vi "Pre-Build Action.vi"(6 "Top Level/Always Included VIs":path[](array[path]), 7 "Main Destination Path":path, 9 "Target Name":string, 10 "Build Specification Name":string, 11 "Project Path":path) -> (0 "error out":errorcluster)   [LabVIEW 2020]
doc: "Get all of the VIPM packages installed in the machine and modify the constant array value to list all installed VIPM packages."
uses:
  <vilib>/JKI/VIPM API/VIPM API_vipm_api.lvlib
panel:
  # "Overview: Get all of the VIPM packages installed in the machine and modify the constant array value to list all installed VIPM packages.\nRequirements: Target VI\nInstructions:\n1. (#TODO1) In the block diagram, specify the target VI reference\n2. (#TODO2) Specify the label name like this in the target VI\nor change the string constant in the block diagram to make it the same as the constant label in the target VI\n(Note: the constant must be 1D String Array)\n3. (#TODO3) Replace the included control/indicator with your orginal control/indicator if you're using the pre-built VI template \n3. Set this VI as Pre Build in the project Build Specifications Properties (Pre/Post Build Actions -> Execute VI before build)"
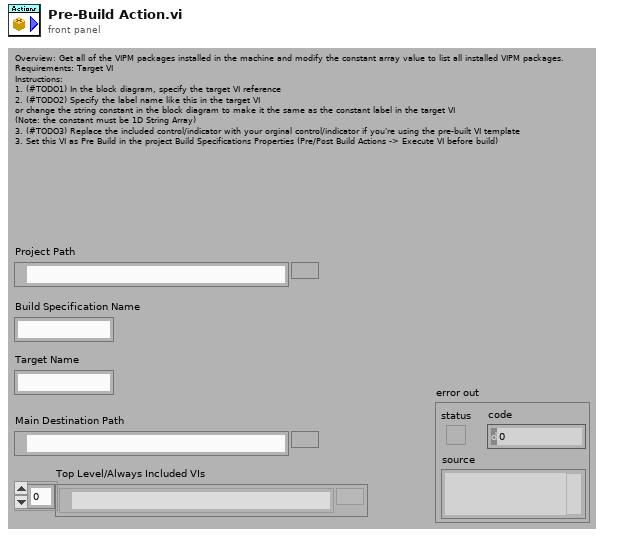
[diagram p1: front panel]
types:
  T1 = typedef "VIPM API_vipm_api.lvlib/LabVIEW Target Info Cluster_vipm_api.ctl" = cluster{"Version":string, "Connection Tested":bool, "Disabled":bool}
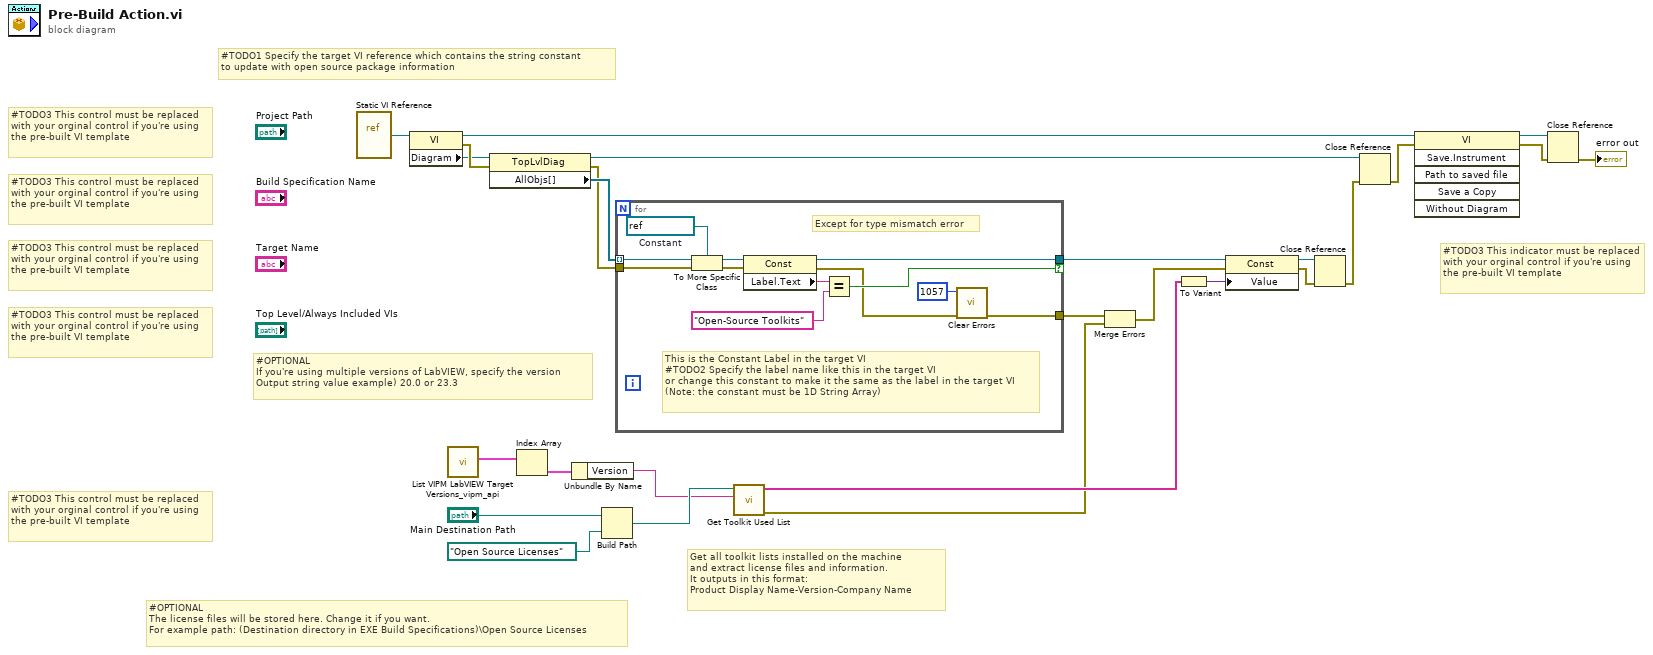
[diagram p0: block diagram]
diagram:
  # "#TODO3 This indicator must be replaced with your orginal control if you're using the pre-built VI template"
  # "#TODO3 This control must be replaced with your orginal control if you're using the pre-built VI template"
  # "#TODO3 This control must be replaced with your orginal control if you're using the pre-built VI template"
  # "#TODO3 This control must be replaced with your orginal control if you're using the pre-built VI template"
  # "#TODO3 This control must be replaced with your orginal control if you're using the pre-built VI template"
  # "#TODO3 This control must be replaced with your orginal control if you're using the pre-built VI template"
  # "Get all toolkit lists installed on the machine\nand extract license files and information.\nIt outputs in this format:\nProduct Display Name-Version-Company Name"
  # "#OPTIONAL\nIf you're using multiple versions of LabVIEW, specify the version\nOutput string value example) 20.0 or 23.3"
  # "#TODO1 Specify the target VI reference which contains the string constant\nto update with open source package information"
  # "#OPTIONAL\nThe license files will be stored here. Change it if you want.\nFor example path: (Destination directory in EXE Build Specifications)\\Open Source Licenses"
  n1 = vi-ref "Static VI Reference"() -> ("vi reference"=w1:refnum<vi>)
  n2 = property class="VI"(reference=w1) -> (reference out=w18:refnum<vi>, error out=w20:errorcluster, "Diagram"=w19:refnum<vi>)  [unwired: 1 in]
  n3 = call <vilib>:"List VIPM LabVIEW Target Versions_vipm_api.vi"() -> ("LabVIEW Target Info"=w8:T1[])  [unwired: 10 in, 1 out]
  n4 = property class="TopLvlDiag"(reference=w19, error in=w20) -> (reference out=w12:refnum<vi>, error out=w17:errorcluster, "AllObjs[]"=w23:refnum<vi>[])
  n5 = Index Array(array=w8) -> (element=w26:T1)  [unwired: 1 in]
  n6 = Unbundle By Name(w26) -> ("Version"=w6:string)
  n7 = Build Path(base path="Main Destination Path", name or relative path=path "Open Source Licenses") -> (appended path=w7:path)
  n8 = for {
    tunnel: w23 -> [w38] mode=indexing
    tunnel: [w34] -> w22 if=w33
    tunnel: w17 -> [w31]
    tunnel: [w28] -> w4
    w37 = refnum<vi> refnum  # Constant
    # "This is the Constant Label in the target VI\n#TODO2 Specify the label name like this in the target VI\nor change this constant to make it the same as the label in the target VI\n(Note: the constant must be 1D String Array)"
    # "Except for type mismatch error"
    n9 = To More Specific Class(target class=w37, reference=w38, error in=w31) -> (specific class reference=w36:refnum<vi>, error out=w30:errorcluster)
    n10 = property class="Const"(reference=w36, error in=w30) -> (reference out=w34:refnum<vi>, error out=w29:errorcluster, "Label.Text"=w35:string)
    n11 = Equal?(x=w35, y="Open-Source Toolkits") -> (x = y?=w33:bool)
    n12 = call <vilib>:"Clear Errors.vi"("error in (no error)"=w29, "specific error code to clear (0: all)"=1057) -> ("error out"=w28:errorcluster)  [unwired: 4 in, 1 out]
  }
  n13 = call "Get Toolkit Used List.vi"("Version"=w6, "Exe License Path"=w7) -> ("error out"=w3:errorcluster, "Open Source Toolkit Used"=w5:string[])  [unwired: 8 in]
  n14 = Merge Errors(w4, w3) -> (w2:errorcluster)
  n15 = To Variant(anything=w5) -> (Variant=w21:variant)
  n16 = property class="Const"(reference=w22, error in=w2, "Value"=w21) -> (reference out=w16:refnum<vi>, error out=w15:errorcluster)
  n17 = Close Reference(reference=w16, error in (no error)=w15) -> (error out=w11:errorcluster)
  n18 = Close Reference(reference=w12, error in (no error)=w11) -> (error out=w10:errorcluster)
  n19 = invoke class="VI" method="Save.Instrument"(reference=w18, error in=w10) -> (reference out=w14:refnum<vi>, error out=w13:errorcluster)  [unwired: 4 in, 4 out]
  n20 = Close Reference(reference=w14, error in (no error)=w13) -> (error out=→"error out":errorcluster)
